vi "Status Reference.vi"(0 "INL DNL Test in":refnum<class "INL DNL Test.lvclass">, 11 "Error in":errorcluster) -> (4 "INL DNL Test out":refnum<class "INL DNL Test.lvclass">, 6 "VI ref":refnum<vi>, 15 "Error out":errorcluster)   [LabVIEW 2020, in "INL DNL Test.lvclass"]
doc: "Runs the status page asynchronously."
uses:
  INL DNL Test.lvclass
  Parent/Typedef/LV2 Control.ctl
  Status Page.vi
  Parent/Test.lvclass
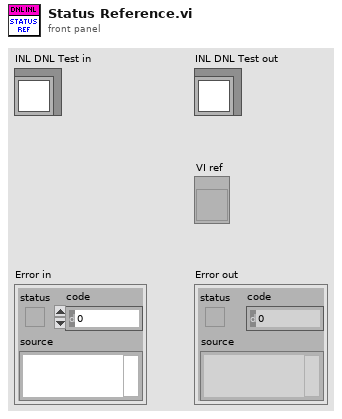
[diagram p1: front panel]
types:
  T1 = typedef "Test.lvclass/LV2 Control.ctl" = enum16{"Home", "Mode", "Config", "Status", "Read"}
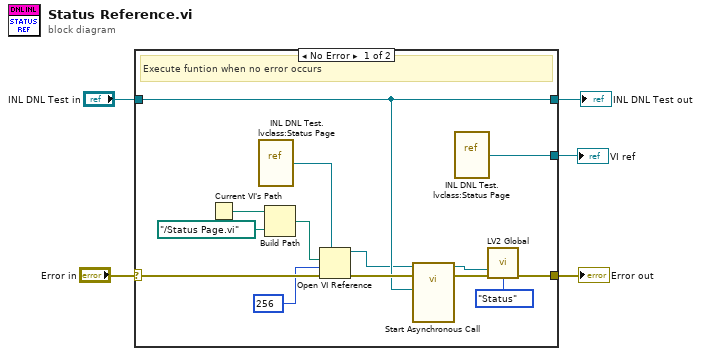
[diagram p0: block diagram]
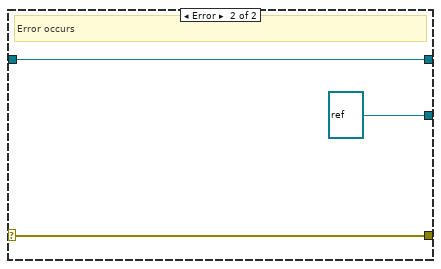
[diagram p2: hidden frame]
diagram:
  n1 = case shown="No Error" "Error in" {
    selector: "Error in" -> [w19 w21]
    tunnel: [w7 w21] -> w4
    tunnel: [w12 w22] -> w2
    tunnel: "INL DNL Test in" -> [w12 w22]
    tunnel: [w18 refnum<vi> refnum] -> w1
    frame No Error {
      # "Execute funtion when no error occurs"
      n2 = Current VI's Path() -> (path=w17:path)
      n3 = vi-ref "INL DNL Test.lvclass:Status Page.vi"() -> (w14:refnum<vi>)
      n4 = Build Path(base path=w17, name or relative path=path "../Status Page.vi") -> (appended path=w15:path)
      n5 = Open VI Reference(type specifier VI Refnum (for type only)=w14, vi path=w15, options=256, error in (no error)=w19) -> (vi reference=w11:refnum<vi>, error out=w13:errorcluster)  [unwired: 2 in]
      n6 = call-by-ref "Start Asynchronous Call"(reference=w11, error in=w13, "INL DNL Test in"=w12) -> (reference out=w9:refnum<vi>, error out=w8:errorcluster)  [unwired: 9 in, 2 out]
      n7 = vi-ref "INL DNL Test.lvclass:Status Page.vi"() -> (w18:refnum<vi>)
      n8 = call "LV2 Global.vi"("Status Ref In"=w9, "Error In"=w8, "Enum"=LV2_Control."Status") -> ("Error Out"=w7:errorcluster)  [unwired: 8 in, 4 out]
    }
    frame Error {
      # "Error occurs"
    }
  }
  "Error out" <- w4
  "INL DNL Test out" <- w2
  "VI ref" <- w1
